vi "process diagnostic data.vi"(7 "expected slave":i8, 8 "error in":errorcluster, 10 "error specs":T1[](array[typedef]), 11 "diagnostic bytes":u8[](array[numeric]) format="%.0b") -> (0 "error out":errorcluster)   [LabVIEW 2013, in "Profibus Module runtime.lvclass"]
uses:
  Profibus Module runtime.lvclass
  configuration/error throw specification.ctl
  configuration/Profibus Module configuration.lvclass
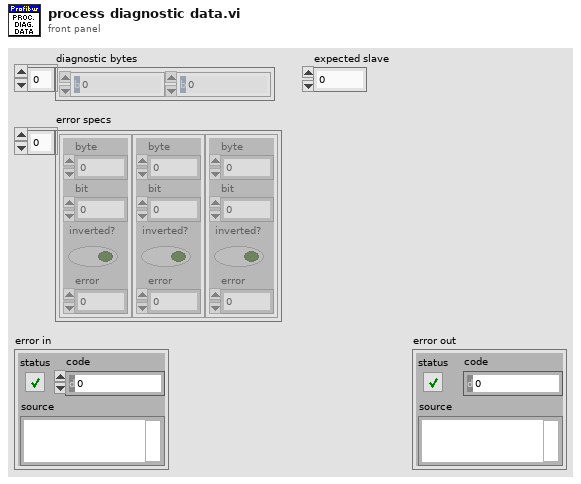
[diagram p1: front panel]
types:
  T1 = typedef "Profibus Module configuration.lvclass/error throw specification.ctl" = cluster{"byte":i32, "bit":i32, "inverted?":bool, "error":i32}
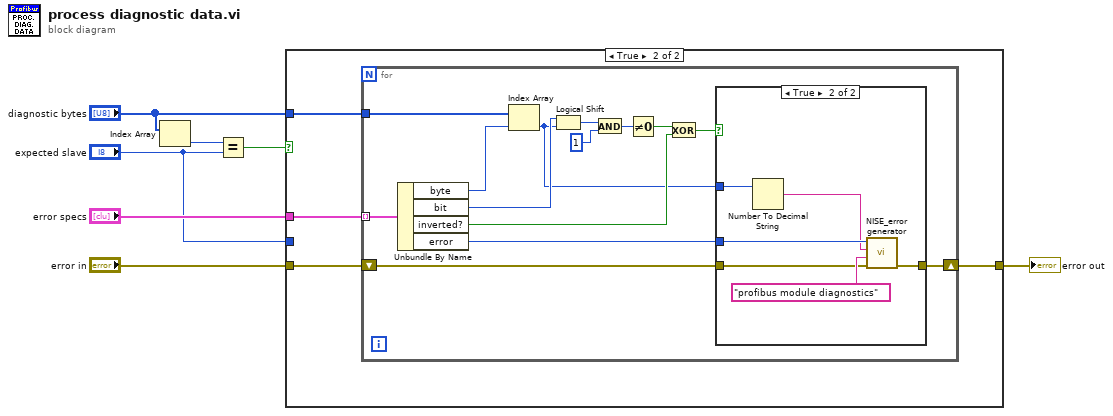
[diagram p0: block diagram]
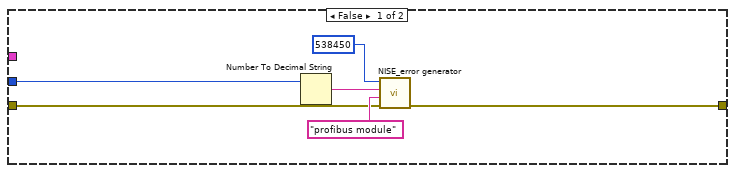
[diagram p2: hidden frame]
diagram:
  n1 = Index Array(array="diagnostic bytes") -> (element=w5:u8)  [unwired: 1 in]
  n2 = Equal?(x=w5, y="expected slave") -> (x = y?=w4:bool)
  n3 = case shown="True" w4 {
    tunnel: "error specs" -> [_ w17]
    tunnel: "diagnostic bytes" -> [_ w16]
    tunnel: [w10 w14] -> w3
    tunnel: "error in" -> [w9 w15]
    tunnel: "expected slave" -> [w8 _]
    frame False {
      n4 = Number To Decimal String(number=w8) -> (decimal integer string=w12:string)  [unwired: 1 in]
      n5 = call <vilib>:"NISE_error generator.vi"("error in"=w9, "source"="profibus module", "append error message"=w12, "error code (0)"=538450) -> ("error out"=w10:errorcluster)  [unwired: 5 in]
    }
    frame True {
      n6 = for {
        tunnel: w17 -> [w31] mode=indexing
        tunnel: w16 -> [w30]
        shift-right: [w19] -> w14
        shift-left: w15 -> [w20]
        n7 = Unbundle By Name(w31) -> ("byte"=w29:i32, "bit"=w28:i32, "inverted?"=w23:bool, "error"=w21:i32)
        n8 = Index Array(array=w30, index=w29) -> (element=w18:u8)
        n9 = Logical Shift(y=w28, x=w18) -> (x << y=w27:u8)
        n10 = And(x=w27, y=u8 1) -> (x .and. y?=w25:u8)
        n11 = Not Equal To 0?(x=w25) -> (x != 0?=w24:bool)
        n12 = Exclusive Or(1:w23, 2:w24) -> (0:w22:bool)
        n13 = case shown="True" w22 {
          tunnel: w21 -> [_ w35]
          tunnel: w20 -> [w32 w37]
          tunnel: [w32 w36] -> w19
          tunnel: w18 -> [_ w34]
          frame False {
          }
          frame True {
            n14 = Number To Decimal String(number=w34) -> (decimal integer string=w33:string)  [unwired: 1 in]
            n15 = call <vilib>:"NISE_error generator.vi"("error in"=w37, "source"="profibus module diagnostics", "append error message"=w33, "error code (0)"=w35) -> ("error out"=w36:errorcluster)  [unwired: 5 in]
          }
        }
      }
    }
  }
  "error out" <- w3
